vi "Save Copy Lib As.vi"(6 "Extension":string=".lvlib", 7 "Application in":refnum<vi>, 8 "error in (no error)":errorcluster, 9 "New Name":string, 10 "Path to Lib Being Copied":path, 11 "Project In":refnum<vi>) -> (0 "error out":errorcluster, 1 "New Lib Ref":refnum<vi>, 2 "New Module/Lib Name":string caption="Name", 3 "New Path":path)   [LabVIEW 2015, in "Generic Module Library.lvlib"]
uses:
  Generic Module Library.lvlib
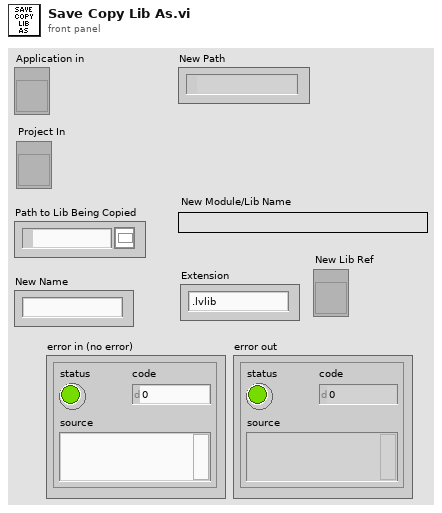
[diagram p1: front panel]
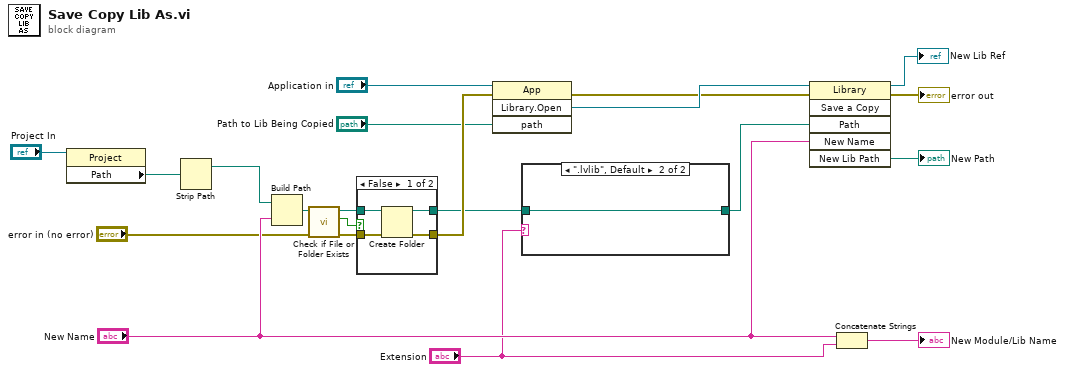
[diagram p0: block diagram]
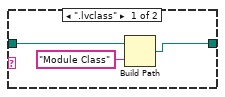
[diagram p2: hidden frame]
diagram:
  n1 = property class="Project"(reference="Project In") -> ("Path"=w2:path)  [unwired: 1 in, 2 out]
  n2 = Strip Path(path=w2) -> (stripped path=w1:path)  [unwired: 1 out]
  n3 = Build Path(base path=w1, name or relative path="New Name") -> (appended path=w15:path)
  n4 = call <vilib>:"Check if File or Folder Exists.vi"("error in (no error)"="error in (no error)", "path"=w15) -> ("error out"=w16:errorcluster, "file or folder exists?"=w18:bool, "dup path"=w17:path)  [unwired: 7 in]
  n5 = case shown="False" w18 {
    tunnel: w16 -> [w25 w26]
    tunnel: w17 -> [w24 w27]
    tunnel: [w22 w27] -> w8
    tunnel: [w23 w26] -> w13
    frame False {
      n6 = Create Folder(path (use dialog)=w24, error in=w25) -> (created path=w22:path, error out=w23:errorcluster)  [unwired: 1 in, 1 out]
    }
    frame True {
    }
  }
  n7 = invoke on="Invoke Node" class="App" method="Library.Open"(reference="Application in", error in=w13, "path"="Path to Lib Being Copied") -> (error out=w12:errorcluster, "Open Library"=w19:refnum<vi>)  [unwired: 1 in, 2 out]
  n8 = case shown="\".lvlib\", Default" "Extension" {
    tunnel: w8 -> [w30 w31]
    tunnel: [w28 w31] -> w7
    frame ".lvclass" {
      n9 = Build Path(base path=w30, name or relative path="Module Class") -> (appended path=w28:path)
    }
    frame ".lvlib", Default {
    }
  }
  n10 = invoke on="Invoke Node" class="Library" method="Save a Copy"(reference=w19, error in=w12, "Path"=w7, "New Name"="New Name") -> (reference out=→"New Lib Ref":refnum<vi>, error out=→"error out":errorcluster, "New Lib Path"=→"New Path":path)  [unwired: 2 in, 3 out]
  n11 = Concatenate Strings("New Name", "Extension") -> (→"New Module/Lib Name":string)
